vi "motion_variables.vi"() -> (2 "Motion variables":T1={"Motion command"="\\\\192.168.1.10\\motion_vars\\Motion command", "Motion status"="\\\\192.168.1.10\\motion_vars\\Motion status", "Emergency stop"="\\\\192.168.1.10\\motion_vars\\Emergency stop", "End transform"="\\\\192.168.1.10\\motion_vars\\End transform", "Home position"="\\\\192.168.1.10\\motion_vars\\Home position", "Axis offsets"="\\\\192.168.1.10\\motion_vars\\Axis offsets"})   [LabVIEW 2013]
uses:
  motion_variables.ctl
panel:
  # "This VI exists to provide a single place that establishes the datasocket associations to the motion server interface.  Except not really, because motion_ui.vi uses control bindings too.  Motion clients should use the accessor VIs with the same name as the variable or one of the higher-level client VIs such as move_to.vi."
  # "Note: to get it so that shared variables on motion server can be accessed from RT target, the shared variable manager must be bound to the RT interface on the motion server machine, see \"Deploying Shared Variables to a Specific Network Card\".  Also the RT target must have datasocket installed.\n\nThe windows firewall on the motion server machine must be configured to allow access.  This procedure worked for me:\n______________________\nGetting the LabVIEW 2011 Shared Variable Server to work through Windows Firewall on Windows 7 x64 will require allowing the following programs to pass through the firewall:\n\nC:\\Windows\\SysWOW64\\lkads.exe\nC:\\Windows\\SysWOW64\\lktsrv.exe\nc:\\Program Files (x86)\\National Instruments\\Shared\\Tagger\\tagsrv.exe\n\nNote: even when using LabVIEW 64-bit, the directory for tagsrv.exe is still under the x86 Program Files.\nNote: For 32 bit windows, the lkads.exe and lktsrv.exe will be under c:\\Windows\\System32\\\n\nAlso, you must allow the following ports through Windows Firewall:\nTCP: 2343, 59110-59115\nUDP: 2343, 6000-6010\n\nFor the TCP ports, you must open one port above 59110 per “per application,”–by opening 59110-59115, we assume that no more than 5 applications are running concurrently.\n_______________________"
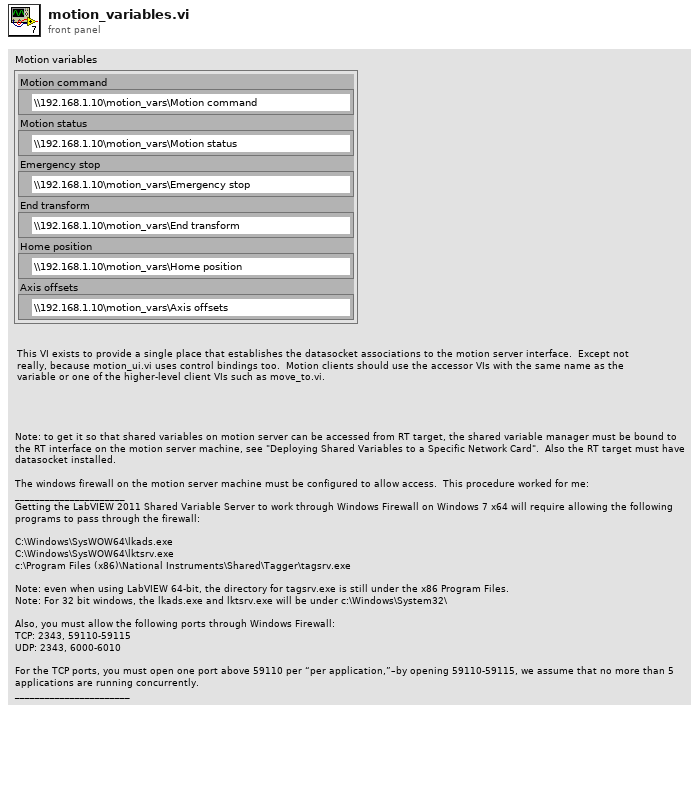
[diagram p1: front panel]
types:
  T1 = typedef "motion_variables.ctl" = cluster{"Motion command":refnum<k21>, "Motion status":refnum<k21>, "Emergency stop":refnum<k21>, "End transform":refnum<k21>, "Home position":refnum<k21>, "Axis offsets":refnum<k21>}
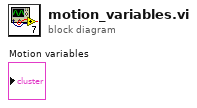
[diagram p0: block diagram]
diagram:
